vi "CalculateTubeLength.vi"(6 "Range":dbl, 8 "Long Tube":dbl, 9 "Mid Tube":dbl, 10 "Short Tube":dbl, 11 "Collar":dbl) -> (3 "Tube Length":dbl)   [LabVIEW 2019]
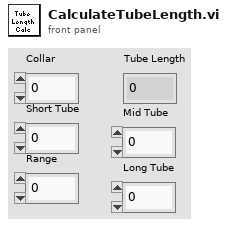
[diagram p1: front panel]
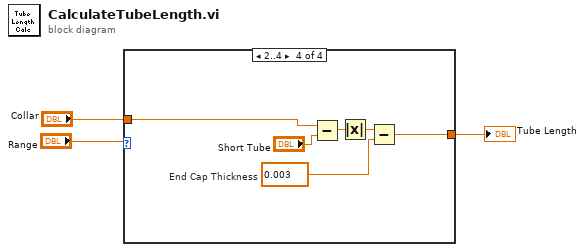
[diagram p0: block diagram]
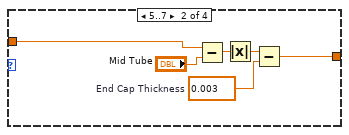
[diagram p3: hidden frame]
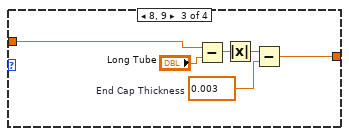
[diagram p4: hidden frame]
diagram:
  n1 = case shown="2..4" "Range" {
    tunnel: [_ w7 w13 w19] -> w3
    tunnel: "Collar" -> [_ w5 w11 w17]
    frame 0, Default {
    }
    frame 5..7 {
      w9 = 0.003  # End Cap Thickness
      n2 = Subtract(x=w5, y="Mid Tube") -> (x-y=w6:dbl)
      n3 = Absolute Value(x=w6) -> (abs(x)=w8:dbl)
      n4 = Subtract(x=w8, y=w9) -> (x-y=w7:dbl)
    }
    frame 8, 9 {
      w15 = 0.003  # End Cap Thickness
      n5 = Subtract(x=w11, y="Long Tube") -> (x-y=w12:dbl)
      n6 = Absolute Value(x=w12) -> (abs(x)=w14:dbl)
      n7 = Subtract(x=w14, y=w15) -> (x-y=w13:dbl)
    }
    frame 2..4 {
      w21 = 0.003  # End Cap Thickness
      n8 = Subtract(x=w17, y="Short Tube") -> (x-y=w18:dbl)
      n9 = Absolute Value(x=w18) -> (abs(x)=w20:dbl)
      n10 = Subtract(x=w20, y=w21) -> (x-y=w19:dbl)
    }
  }
  "Tube Length" <- w3
